vi "LIA Simulation 48 Bits Slicer.vi"() -> ()   [LabVIEW 2017]
panel:
  out "fixed-point 3":fxp<+/-,22,2> format="%.0x"
  out "fixed-point 2":fxp<+/-,22,2> format="%.0x"
  in  "fixed-point":fxp<+,48,48> format="%.0b"
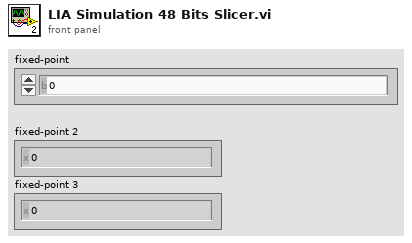
[diagram p1: front panel]
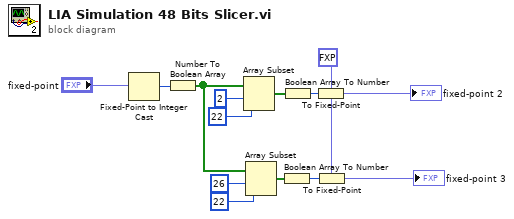
[diagram p0: block diagram]
diagram:
  w3 = fxp<+/-,22,2> 0.0 ("fixed-point type")
  n1 = Fixed-Point to Integer Cast(1:"fixed-point") -> (0:w14:u64)
  n2 = Number To Boolean Array(number=w14) -> (Boolean array=w12:bool[])
  n3 = Array Subset(array=w12, index=2, length=22) -> (w7:bool[])
  n4 = Array Subset(array=w12, index=26, length=22) -> (w6:bool[])
  n5 = Boolean Array To Number(Boolean array=w6) -> (number=w4:u32)
  n6 = Boolean Array To Number(Boolean array=w7) -> (number=w5:u32)
  n7 = To Fixed-Point(fixed-point type=w3, number=w5) -> (fixed-point=→"fixed-point 2":fxp<+/-,22,2>)
  n8 = To Fixed-Point(fixed-point type=w3, number=w4) -> (fixed-point=→"fixed-point 3":fxp<+/-,22,2>)
